vi "re_do_script_lua.vi"(5 "LuaVIEW reference":T1) -> (15 "error out":errorcluster)   [LabVIEW 2012]
doc: "Call the \"Do Script\" API VI to compile and execute a script. The script is given its own virtual machine instance. This implies that it does not share variables with the script calling this function.\n\nSince LabVIEW has problems with recursion, it is not possible to call <code>do_script()</code> from inside a script started via <code>do_script()</code>. In such a case, the error message result will contain a LabVIEW recursion error. To do a do from a do, the thing to do is to copy the do function VI and rename it to, say, do2 and call into that do too. Note that <code>do_task()</code> does not suffer from this limitation since the creation of a top-level context causes a discontinuity in the call chain.\n\nBy calling this function through <code>lv.pcall()</code>, you can execute a bit of code that can throw errors or has other ill-defined behaviour without risking the termination of your script or the corruption of its variable space.\n\nIf the script is contained in a file, a relative path or bare filename will be resolved by searching relative to the configured script search directories. If no script search directories are configured, the resource base path is searched. If this function is called from a task context, the directory holding the main script of the calling task is searched first.\nParameters:\nstr:name, when the optional script string is not specified, this is the filename plus any path from which to load the script. Otherwise it is the name used to refer to the script when reporting errors.\n[str:script], optional script string allows direct specification of a bit of Lua code. It is advisable to make it a literal string by enclosing it in double square brackets.\nErrors:\nCould not load script.\nScript compilation error.\nLabVIEW recursion error.\nAny error thrown while executing the script."
uses:
  typedefs/t_LuaVIEW Reference.ctl
  subvis/private/LuaVIEW Pull (path).vi
  subvis/private/LuaVIEW Pull (string).vi
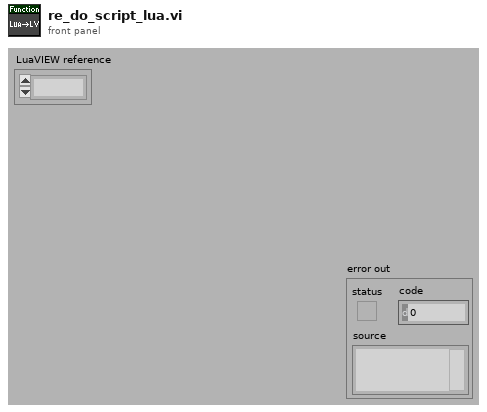
[diagram p1: front panel]
types:
  T1 = typedef "t_LuaVIEW Reference.ctl" = refnum<k1>
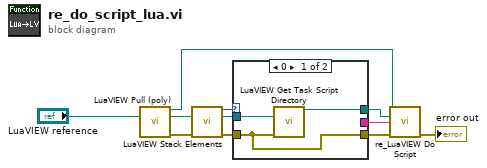
[diagram p0: block diagram]
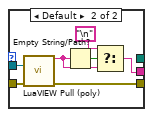
[diagram p2: hidden frame]
diagram:
  n1 = call-poly "LuaVIEW Pull (poly).vi"("LuaVIEW reference in"="LuaVIEW reference") -> ("path"=w1:path, "LuaVIEW reference out"=w9:T1, "error out"=w10:errorcluster)  [unwired: 12 in]
  n2 = call "LuaVIEW Stack Elements.vi"("LuaVIEW reference in"=w9, "error in (no error)"=w10) -> ("elements"=w8:i32, "LuaVIEW reference out"=w5:T1, "error out"=w7:errorcluster)  [unwired: 11 in]
  n3 = case shown="0" w8 {
    tunnel: w7 -> [w14 w21]
    tunnel: [w14 w20] -> w3
    tunnel: [_ w19] -> w6
    tunnel: w5 -> [w12 w15]
    tunnel: [w13 _] -> w4
    frame 0 {
      n4 = call "LuaVIEW Get Task Script Directory.vi"("LuaVIEW reference in"=w12, "error in (no error)"=w14) -> ("task script directory"=w13:path)  [unwired: 11 in, 2 out]
    }
    frame Default {
      n5 = call-poly "LuaVIEW Pull (poly).vi"("LuaVIEW reference in"=w15, "error in (no error)"=w21) -> ("string"=w17:string, "error out"=w20:errorcluster)  [unwired: 11 in, 1 out]
      n6 = Empty String/Path?(string/path=w17) -> (empty?=w18:bool)
      n7 = Select(t="\n", s=w18, f=w17) -> (s? t:f=w19:string)
    }
  }
  n8 = call "re_LuaVIEW Do Script.vi"("script file or name (no name)"=w1, "custom search directory (none)"=w4, "script string (\"\" == load from file)"=w6, "error in (no error)"=w3) -> ("error out"=→"error out":errorcluster)  [unwired: 11 in]
